vi "Read Protected Event.vi"(8 "error in (no error)":errorcluster, 11 "0MQ_Server in":refnum<class "0MQ_Server.lvclass">) -> (0 "error out":errorcluster, 2 "Protected Events":T1, 3 "0MQ_Server out":refnum<class "0MQ_Server.lvclass">)   [LabVIEW 2016, in "0MQ_Server.lvclass"]
uses:
  0MQ_Server.lvclass
  Typedefs/0MQ_Server.ProtectedEvents.ctl
  0MQ_Server.lvclass/0MQ_Server.ctl
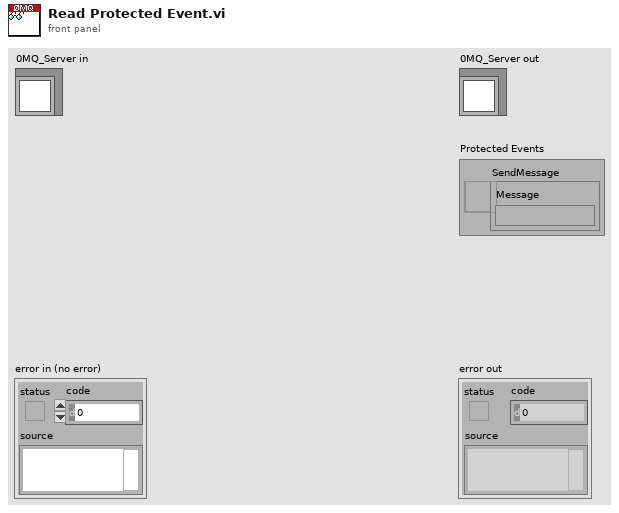
[diagram p1: front panel]
types:
  T1 = typedef "0MQ_Server.lvclass/0MQ_Server.ProtectedEvents.ctl" = cluster{"SendMessage":refnum<user-event>}
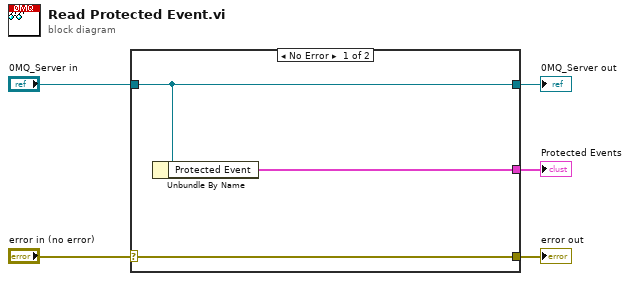
[diagram p0: block diagram]
diagram:
  n1 = case shown="No Error" "error in (no error)" {
    selector: "error in (no error)" -> [w8 w9]
    tunnel: [w8 w9] -> w4
    tunnel: [w7 w10] -> w2
    tunnel: "0MQ_Server in" -> [w7 w10]
    tunnel: [w6 _] -> w1
    frame No Error {
      n2 = Unbundle By Name(w7) -> ("Protected Event"=w6:T1)
    }
    frame Error {
    }
  }
  "error out" <- w4
  "0MQ_Server out" <- w2
  "Protected Events" <- w1
